vi "Main.vi"() -> ()   [LabVIEW 2021]
uses:
  <vilib>/MakerHub/LINX/Public/Peripherals/Digital/Digital Write 1 Chan.vi
  <vilib>/MakerHub/LINX/Public/Peripherals/Digital/Digital Write N Chans.vi
  <vilib>/MakerHub/LINX/Private/Local IO/LinxDigitalWrite.vi
  <vilib>/MakerHub/LINX/Public/Utilities/Check Channel.vi
  <vilib>/MakerHub/LINX/Private/Local IO/Handle Errors.vi
  <vilib>/LabVIEW Open Source Project/Connection/Connection.TCP/Connection.TCP.lvclass
  C:/Program Files (x86)/National Instruments/LabVIEW 2021/vi.lib/LabVIEW Open Source Project/Connection/Connection/Connection.lvclass
  <vilib>/LabVIEW Open Source Project/MQTT Client/Client class/Client.lvclass
  C:/Program Files (x86)/National Instruments/LabVIEW 2021/vi.lib/LabVIEW Open Source Project/MQTT Connection/MQTT_Base/Base Class/MQTT_Base.lvclass
  <vilib>/Plasmionique/MB Master/MB_Master_Serial/MB_Master_Serial.lvclass
  C:/Program Files (x86)/National Instruments/LabVIEW 2021/vi.lib/Plasmionique/MB Master/MB_Master/MB_Master.lvclass
  <vilib>/MakerHub/LINX/Public/Utilities/Open Local.vi
  <vilib>/MakerHub/LINX/Private/Utilties/Generate Error.vi
  <vilib>/Plasmionique/MB Master/MB Master.lvlib
  <vilib>/MakerHub/LINX/LMH-LINX.lvlib
  <vilib>/LabVIEW Open Source Project/MQTT Connection/MQTT_Base/Base Class/MQTT_Base.lvclass
  <vilib>/LabVIEW Open Source Project/Connection/Connection.LocalQueue/Connection.LocalQueue.lvclass
  <vilib>/LabVIEW Open Source Project/Connection/Connection/Connection.lvclass
panel:
  out "JSON string":string
  out "Energia Acumulada":dbl
  out "Potência":dbl
  in  "Stop Client":bool
  out "Published":bool
  out "Connected":bool
  out "Temperatura ºC 2":dbl
  in  "Stop Button":bool
  out "Temperatura ºC":dbl
  out "Tensão":dbl
  out "Corrente":dbl
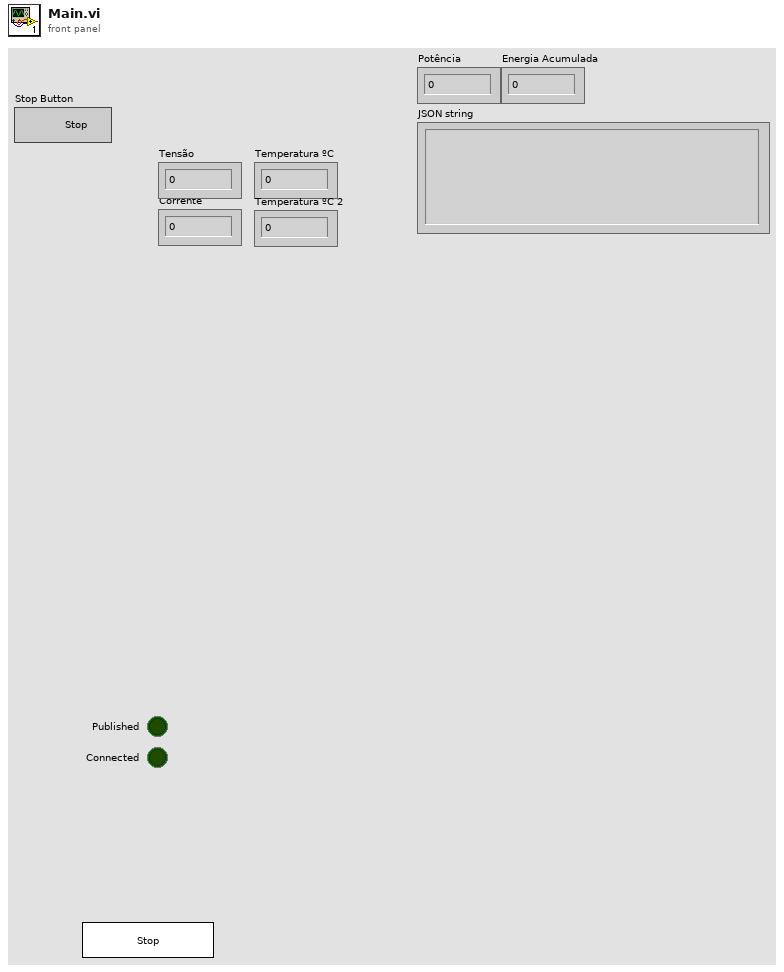
[diagram p1: front panel]
types:
  T1 = cluster{"baud rate (bps)":u32, "stop bits":u16, "parity":u16, "flow control":u16, "timeout":u32, "retries":i32}
  T2 = typedef "LMH-LINX.lvlib/LINX Ref.ctl" = cluster{"IO":T3, "Interface":T4, "LINX Device Config":T5}
  T3 = typedef "LMH-LINX.lvlib/Platform.ctl" = enum16{"Remote", "Local"}
  T4 = typedef "LMH-LINX.lvlib/Interface.ctl" = enum16{"Serial", "TCP"}
  T5 = typedef "LMH-LINX.lvlib/Device.lvlib/LINX Device Config.ctl" = cluster{"Interface":T4, "COM Port":refnum<visa-resource-name>, "TCP Configuration":T6, "Device Family":u8, "Device ID":u8, "Device Name":string, "TCP Ref":refnum<k5>, "Channels":T7}
  T6 = typedef "LMH-LINX.lvlib/Device.lvlib/TCP Config.ctl" = cluster{"IP Address":string, "Port":u16}
  T7 = typedef "LMH-LINX.lvlib/Channels.ctl" = cluster{"DI":u8[], "DO":u8[], "AI":u8[], "AO":u8[], "PWM":u8[], "QE":u8[], "UART":u8[], "I2C 2":u8[], "SPI":u8[], "CAN":u8[], "Servo":u8[], "AI Ref (V)":dbl, "AI Resolution (Bits)":u8, "AO Ref (V)":dbl, "AO Resolution (Bits)":u8}
  T8 = cluster{"Tensao":dbl, "Corrente":dbl, "Potencia":dbl, "Energia":dbl, "Temperatura 1":dbl, "Temperatura 2":dbl}
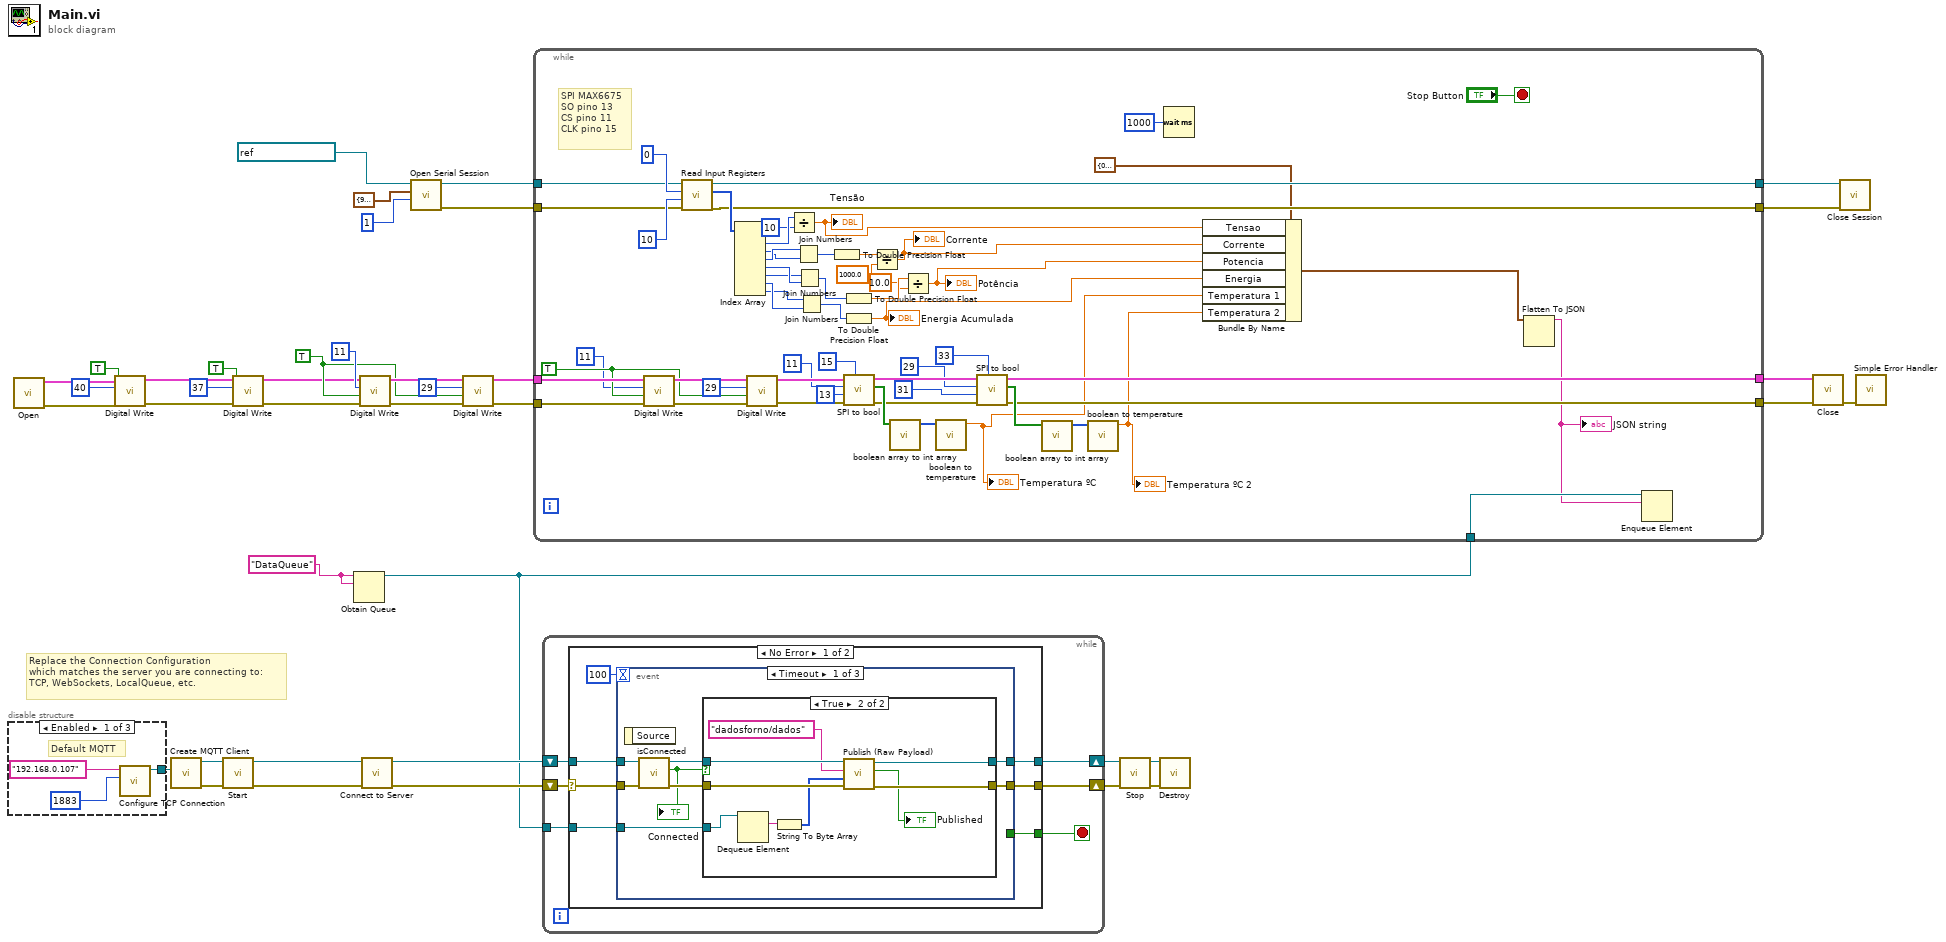
[diagram p0: block diagram]
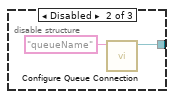
[diagram p2: hidden frame]
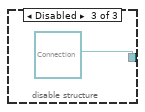
[diagram p3: hidden frame]
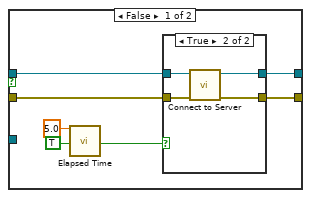
[diagram p4: hidden frame]
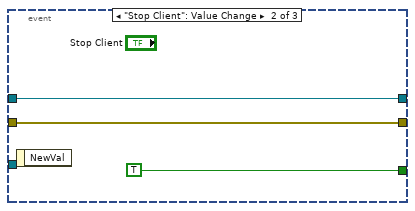
[diagram p6: hidden frame]
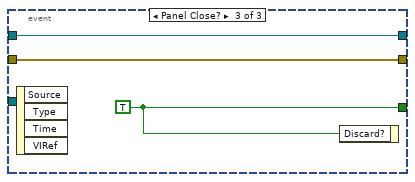
[diagram p7: hidden frame]
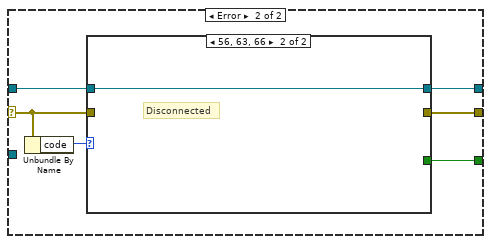
[diagram p8: hidden frame]
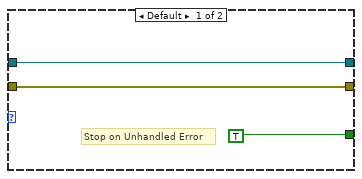
[diagram p9: hidden frame]
diagram:
  w2 = "DataQueue" ("name (unnamed)")
  w25 = TRUE ("Output Value")
  # "Replace the Connection Configuration\nwhich matches the server you are connecting to:\nTCP, WebSockets, LocalQueue, etc."
  n1 = disable-structure shown="Enabled" {
    disable-tunnel: [w42 w45 refnum<class "Connection.lvclass"> refnum ("Connection Configuration")] -> w13
    frame Enabled {
      # "Default MQTT"
      n2 = call <vilib>:"Configure TCP Connection.vi"("remote port (80)"=u16 1883, "address (localhost)"="192.168.0.107") -> ("Connection.TCP"=w42:refnum<class "Connection.TCP.lvclass">)  [unwired: 8 in, 1 out]
    }
    frame Disabled {
      n3 = call <vilib>:"Configure Queue Connection.vi"("Queue Name"="queueName") -> ("Connection.LocalQueue"=w45:refnum<class "Connection.LocalQueue.lvclass">)  [unwired: 9 in, 1 out]
    }
    frame Disabled {
    }
  }
  n4 = call-poly <vilib>:"Open.vi"() -> ("Error Out"=w16:errorcluster, "LINX Resource"=w17:T2)  [unwired: 9 in, 1 out]
  n5 = call-poly <vilib>:"Digital Write.vi"("Error In"=w16, "Output Value"=TRUE, "DO Channel"=u8 40, "LINX Resource"=w17) -> ("Error Out"=w14:errorcluster, "LINX Resource"=w15:T2)  [unwired: 6 in]
  n6 = call <vilib>:"Create MQTT Client.vi"("Connection Configuration"=w13) -> ("error out"=w7:errorcluster, "Client out"=w8:refnum<class "Client.lvclass">)  [unwired: 9 in]
  n7 = call <vilib>:"Start.vi"("error in (no error)"=w7, "MQTT_Base in"=w8) -> ("error out"=w5:errorcluster, "MQTT_Base out"=w6:refnum<class "Client.lvclass">)  [unwired: 7 in, 1 out]
  n8 = call-poly <vilib>:"Digital Write.vi"("Error In"=w14, "Output Value"=TRUE, "DO Channel"=u8 37, "LINX Resource"=w15) -> ("Error Out"=w22:errorcluster, "LINX Resource"=w23:T2)  [unwired: 6 in]
  n9 = Obtain Queue(name (unnamed)=w2, element data type=w2) -> (queue out=w1:refnum<queue>)  [unwired: 3 in, 2 out]
  n10 = call-poly <vilib>:"Digital Write.vi"("Error In"=w22, "Output Value"=w25, "DO Channel"=u8 11, "LINX Resource"=w23) -> ("Error Out"=w28:errorcluster, "LINX Resource"=w29:T2)  [unwired: 6 in]
  n11 = call <vilib>:"Connect to Server.vi"("error in (no error)"=w5, "Client in"=w6) -> ("error out"=w3:errorcluster, "Client out"=w4:refnum<class "Client.lvclass">)  [unwired: 6 in, 2 out]
  n12 = call <vilib>:"Open Serial Session.vi"("Slave ID"=u8 1, "Serial Config"=T1 {"baud rate (bps)"=9600, "stop bits"=10, "parity"=0, "flow control"=0, "timeout"=1000, "retries"=1}, "VISA Resource"=refnum<visa-resource-name> "ASRL1::INSTR") -> ("Error out"=w36:errorcluster, "MB_Serial session"=w37:refnum<class "MB_Master_Serial.lvclass">)  [unwired: 7 in]
  n13 = call-poly <vilib>:"Digital Write.vi"("Error In"=w28, "Output Value"=w25, "DO Channel"=u8 29, "LINX Resource"=w29) -> ("Error Out"=w27:errorcluster, "LINX Resource"=w26:T2)  [unwired: 6 in]
  n14 = while {
    tunnel: w37 -> [w94]
    tunnel: w36 -> [w93]
    tunnel: [w92] -> w35
    tunnel: [w91] -> w34
    tunnel: [w85] -> w31
    tunnel: [w84] -> w30
    tunnel: w26 -> [w79]
    tunnel: w27 -> [w78]
    tunnel: w1 -> [w65]
    stop <- "Stop Button" stop-if-true
    w77 = TRUE ("Output Value")
    # "SPI MAX6675\nSO pino 13\nCS pino 11\nCLK pino 15"
    n15 = call-poly <vilib>:"Digital Write.vi"("Error In"=w78, "Output Value"=w77, "DO Channel"=u8 11, "LINX Resource"=w79) -> ("Error Out"=w81:errorcluster, "LINX Resource"=w80:T2)  [unwired: 6 in]
    n16 = call <vilib>:"Read Input Registers.vi"("error in (no error)"=w93, "quantity"=u16 10, "starting address"=u16 0, "MB session in"=w94) -> ("error out"=w91:errorcluster, "Registers"=w101:u16[], "MB session out"=w92:refnum<class "MB_Master_Serial.lvclass">)  [unwired: 5 in]
    n17 = Index Array(array=w101) -> (element #1=w98:u16, element #2=w99:u16, element #3=w100:u16, element #4=w63:u16, element #5=w62:u16, element #6=w61:u16, element #7=w60:u16)  [unwired: 7 in]
    n18 = call-poly <vilib>:"Digital Write.vi"("Error In"=w81, "Output Value"=w77, "DO Channel"=u8 29, "LINX Resource"=w80) -> ("Error Out"=w75:errorcluster, "LINX Resource"=w76:T2)  [unwired: 6 in]
    n19 = Divide(x=w98, y=u16 10) -> (x/y=w55:dbl)
    "Tensão" <- w55
    n20 = Join Numbers(hi=w100, lo=w99) -> ((hi.lo)=w64:u32)
    n21 = Join Numbers(hi=w62, lo=w63) -> ((hi.lo)=w59:u32)
    n22 = Join Numbers(hi=w60, lo=w61) -> ((hi.lo)=w58:u32)
    n23 = To Double Precision Float(number=w64) -> (double precision float=w96:dbl)
    n24 = To Double Precision Float(number=w59) -> (double precision float=w57:dbl)
    n25 = To Double Precision Float(number=w58) -> (double precision float=w52:dbl)
    "Energia Acumulada" <- w52
    n26 = call "SPI to bool.vi"("SCK"=u8 15, "error in (no error)"=w75, "DO"=u8 13, "SPI CS"=u8 11, "LINX Resource in"=w76) -> ("error out"=w88:errorcluster, "Array"=w90:bool[], "LINX Resource out"=w83:T2)  [unwired: 4 in]
    n27 = Divide(x=w96, y=1000.0) -> (x/y=w54:dbl)
    "Corrente" <- w54
    n28 = call "boolean array to int array.vi"("Array 3"=w90) -> ("Array 2"=w89:u8[])  [unwired: 9 in, 1 out]
    n29 = Divide(x=w57, y=10.0) -> (x/y=w53:dbl)
    "Potência" <- w53
    n30 = call "boolean to temperature.vi"("SPI array"=w89) -> ("Temperatura"=w51:dbl)  [unwired: 10 in]
    "Temperatura ºC" <- w51
    n31 = call "SPI to bool.vi"("SCK"=u8 33, "error in (no error)"=w88, "DO"=u8 31, "SPI CS"=u8 29, "LINX Resource in"=w83) -> ("error out"=w84:errorcluster, "Array"=w86:bool[], "LINX Resource out"=w85:T2)  [unwired: 4 in]
    n32 = call "boolean array to int array.vi"("Array 3"=w86) -> ("Array 2"=w87:u8[])  [unwired: 9 in, 1 out]
    n33 = call "boolean to temperature.vi"("SPI array"=w87) -> ("Temperatura"=w50:dbl)  [unwired: 10 in]
    "Temperatura ºC 2" <- w50
    n34 = Wait (ms)(milliseconds to wait=u32 1000) -> ()  [unwired: 1 out]
    n35 = Bundle By Name(cluster=T8 {"Tensao"=0.0, "Corrente"=0.0, "Potencia"=0.0, "Energia"=0.0, "Temperatura 1"=0.0, "Temperatura 2"=0.0}, "Tensao"=w55, "Corrente"=w54, "Potencia"=w53, "Energia"=w52, "Temperatura 1"=w51, "Temperatura 2"=w50) -> (w48:T8)
    n36 = Flatten To JSON(anything=w48) -> (JSON string=w47:string)  [unwired: 2 in, 1 out]
    "JSON string" <- w47
    n37 = Enqueue Element(queue=w65, element=w47) -> ()  [unwired: 2 in, 3 out]
  }
  n38 = while {
    shift-right: [w107] -> w10
    shift-left: w4 -> [w108]
    shift-right: [w109] -> w12
    shift-left: w3 -> [w105]
    tunnel: w1 -> [w104]
    stop <- w106 stop-if-true
    n39 = case shown="No Error" w105 {
      selector: w105 -> [w111 w153]
      tunnel: [w116 w155] -> w109
      tunnel: w108 -> [w114 w157]
      tunnel: [w113 w156] -> w107
      tunnel: [w112 w154] -> w106
      tunnel: w104 -> [w110 _]
      frame No Error {
        n40 = event shown="[0] Timeout" {
          selector: _ -> [_ _ _]
          dyn-events: _ -> [_ _ _]
          timeout: 100 -> [_ _ _]
          tunnel: w111 -> [w120 w148 w150]
          tunnel: [w123 w148 w150] -> w116
          tunnel: [_ TRUE w152] -> w112
          tunnel: w114 -> [w122 w149 w151]
          tunnel: [w124 w149 w151] -> w113
          tunnel: w110 -> [w117 _ _]
          event Timeout {
            n41 = event-data() -> ()  [unwired: 1 in, 1 out]
            n42 = call <vilib>:"isConnected.vi"("error in (no error)"=w120, "Client in"=w122) -> ("error out"=w119:errorcluster, "connected"=w118:bool, "Client out"=w121:refnum<class "Client.lvclass">)  [unwired: 7 in]
            "Connected" <- w118
            n43 = case shown="True" w118 {
              tunnel: [w130 w144] -> w124
              tunnel: [w128 w143] -> w123
              tunnel: w121 -> [w131 w145]
              tunnel: w119 -> [w129 w146]
              tunnel: w117 -> [_ w140]
              frame False {
                n44 = call "Elapsed Time"("Time Target (s)"=5.0, "Auto Reset"=TRUE) -> ("Time has Elapsed"=w127:bool)  [unwired: 10 in, 7 out]
                n45 = case shown="True" w127 {
                  tunnel: w131 -> [w133 w137]
                  tunnel: [w133 w136] -> w130
                  tunnel: w129 -> [w132 w135]
                  tunnel: [w132 w134] -> w128
                  frame False {
                  }
                  frame True {
                    n46 = call <vilib>:"Connect to Server.vi"("error in (no error)"=w135, "Client in"=w137) -> ("error out"=w134:errorcluster, "Client out"=w136:refnum<class "Client.lvclass">)  [unwired: 6 in, 2 out]
                  }
                }
              }
              frame True {
                n47 = Dequeue Element(queue=w140) -> (element=w139:string)  [unwired: 2 in, 3 out]
                n48 = String To Byte Array(string=w139) -> (unsigned byte array=w138:u8[])
                n49 = call <vilib>:"Publish (Raw Payload).vi"("error in (no error)"=w146, "Binary Payload"=w138, "Topic Name"="dadosforno/dados" ("Topic Name (empty: Payload name)"), "Client in"=w145) -> ("error out"=w143:errorcluster, "Published"=→"Published":bool, "Client out"=w144:refnum<class "Client.lvclass">)  [unwired: 5 in]
              }
            }
          }
          event "Stop Client": Value Change {
            n50 = event-data() -> ()  [unwired: 1 in, 1 out]
          }
          event Panel Close? {
            w152 = TRUE
            n51 = event-data() -> ()  [unwired: 1 in, 4 out]
            n52 = event-data("Discard?"=w152) -> ()  [unwired: 1 in, 1 out]
          }
        }
      }
      frame Error {
        n53 = Unbundle By Name(w153) -> ("code"=w158:i32)
        n54 = case shown="56, 63, 66" w158 {
          tunnel: w157 -> [w161 w162]
          tunnel: [w161 w162] -> w156
          tunnel: w153 -> [w160 _]
          tunnel: [w160 _] -> w155
          tunnel: [TRUE _] -> w154
          frame Default {
            # "Stop on Unhandled Error"
          }
          frame 56, 63, 66 {
            # "Disconnected"
          }
        }
      }
    }
  }
  n55 = call <vilib>:"Stop.vi"("error in (no error)"=w12, "MQTT_Base in"=w10) -> ("error out"=w11:errorcluster, "MQTT_Base out"=w9:refnum<class "Client.lvclass">)  [unwired: 7 in, 1 out]
  n56 = call <vilib>:"Destroy.vi"("error in (no error)"=w11, "MQTT_Base in"=w9) -> ()  [unwired: 8 in, 2 out]
  n57 = call <vilib>:"Close.vi"("Error In"=w30, "LINX Resource"=w31) -> ("Error Out"=w32:errorcluster)  [unwired: 9 in]
  n58 = call-dynamic "Close Session.vi"("error in (no error)"=w34, "MB_Serial session"=w35) -> ()  [unwired: 9 in, 1 out]
  n59 = call <vilib>:"Simple Error Handler.vi"("error in (no error)"=w32) -> ()  [unwired: 4 in, 5 out]
